vi "Set Package Info To VIs - NIPKG.vi"(0 "Project Path":path, 1 "Top Level/Always Included VIs":path[](array[path]), 5 "NIPKG Build Spec Name (NIPKG)":string="NIPKG", 7 "Target Name (My Computer)":string="My Computer", 9 "Destination Path":path, 11 "error in":errorcluster, 12 "Files Generated By Build":path[](array[path])) -> (15 "error out":errorcluster)   [LabVIEW 2017, in "CL_G3_VIComponentBuilder.lvlib"]
doc: "<B>Package details</B>\nVI Component Builder - NIPKG - v1.0.0-21\n\nPackage Filename - vicomponentbuilder-nipkg-1.0.0-21.nipkg"
uses:
  CL_G3_VIComponentBuilder.lvlib
  Exports/NIPKG_LV/NIPKG_LV.lvclass
  <vilib>/LVH/i3 JSON/JSON Parsing/Get Object Parameter Files/Get Object Parameter - Object.vi
  <vilib>/LVH/i3 JSON/JSON Parsing/Get Object Parameter Files/Get Object Parameter - Boolean.vi
  <vilib>/xml/Load XML File.vi
  <vilib>/xml/Close Reference(Node).vi
  <vilib>/xml/NI_XML.lvlib
  <vilib>/LVH/i3 JSON/i3-json.lvlib
panel:
  out "String":string
  out "Progress":i32(slide) scale=-1.0..109.0
  out "Total":i32
  # "Adding Package details to VI description"
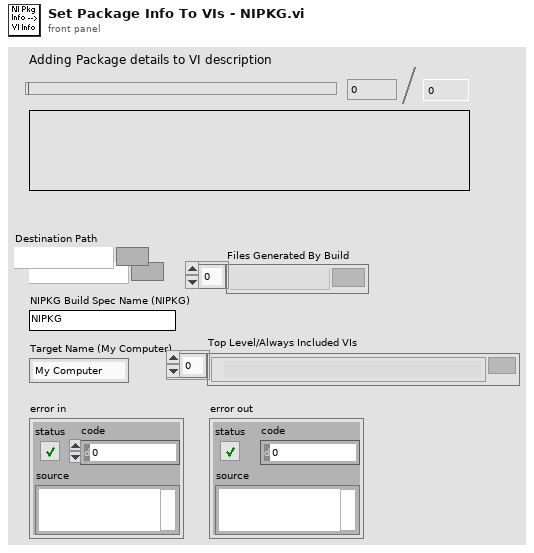
[diagram p1: front panel]
types:
  T1 = cluster{"Error State":errorcluster, "Processed Documentation":string, "Build Spec Path":path, "VIs In Package":path[], "Product Name":string, "Package Version":string, "Package Name":string, "Current File to process":path, "vi reference being processed":refnum<vi>, "Opened References":refnum<vi>[], "Build Options i3JSON Tree":variant}
  T2 = enum32{"Invalid", "Standard", "Closed", "Hidden", "Minimized", "Maximized"}
  T3 = cluster{"Beginning of Tag Position":i32, "End of Tag Position":i32}[]
  T4 = cluster{"Beginning of Tag Position":i32, "End of Tag Position":i32}
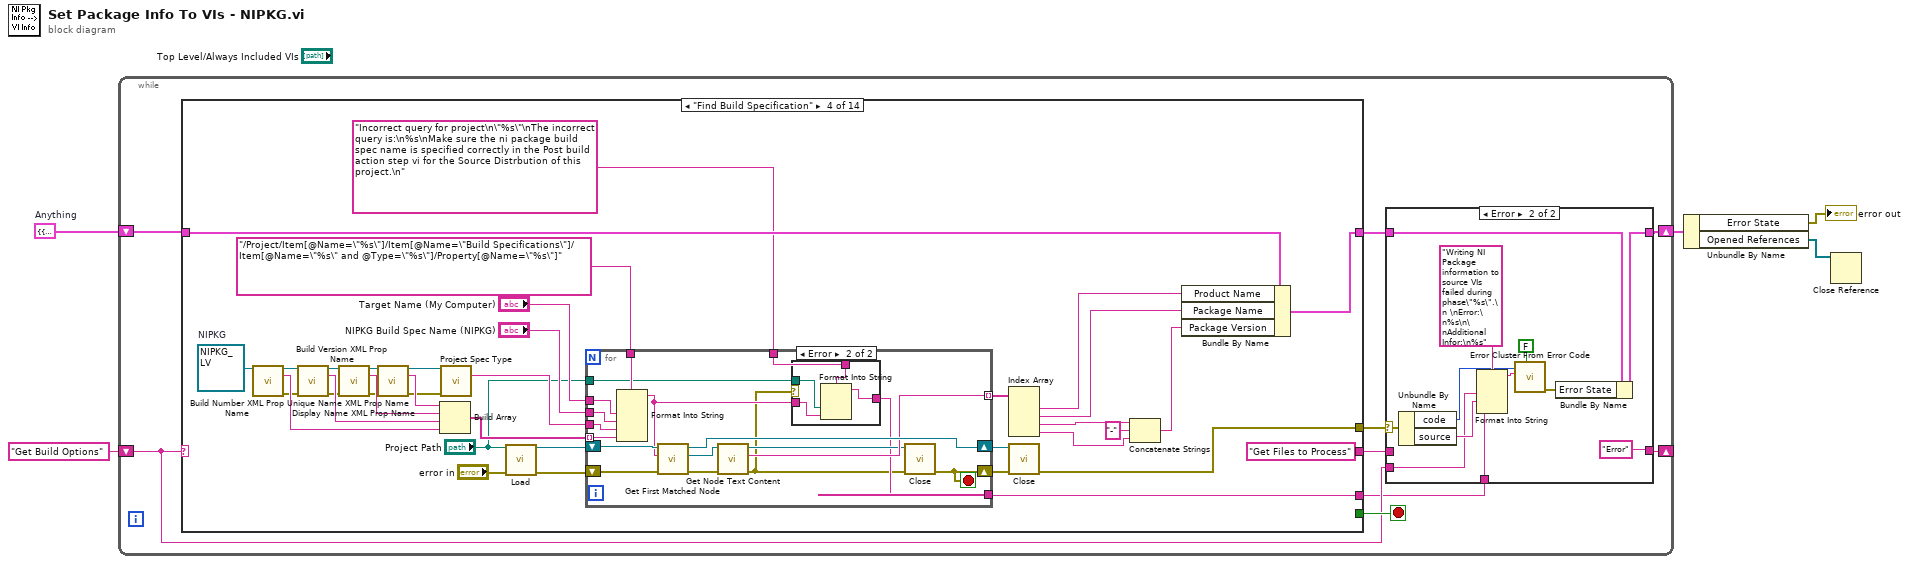
[diagram p0: block diagram]
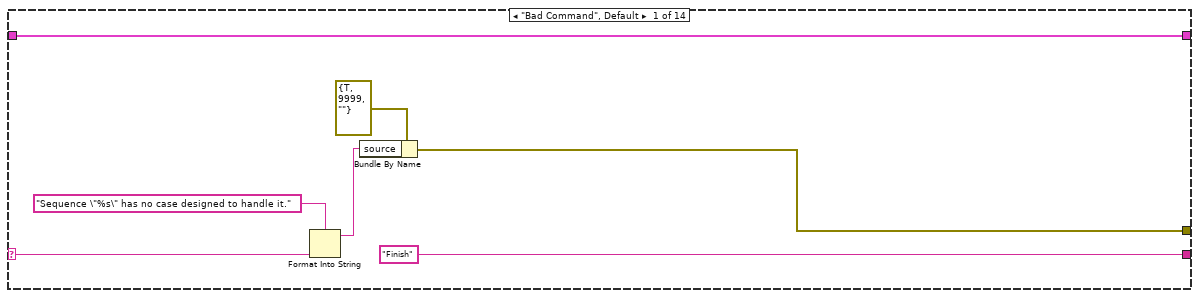
[diagram p3: hidden frame]
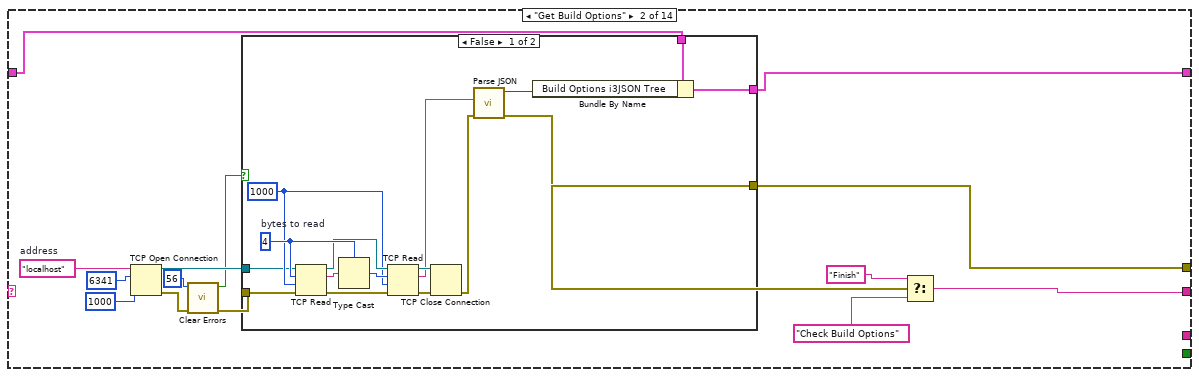
[diagram p4: hidden frame]
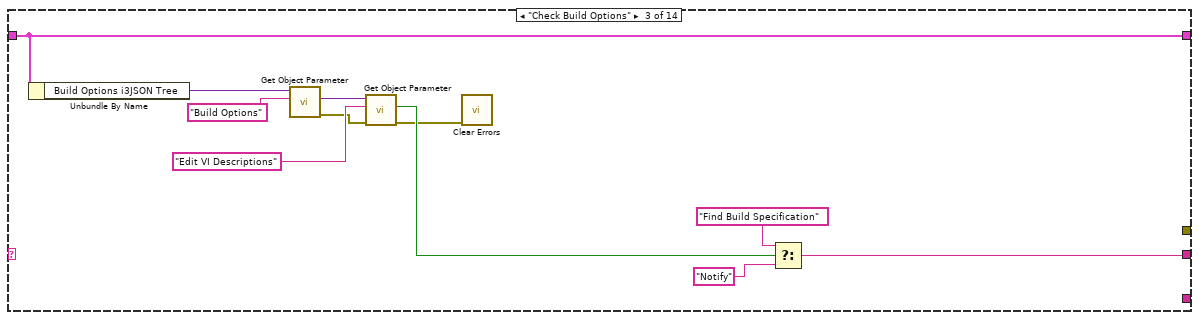
[diagram p6: hidden frame]
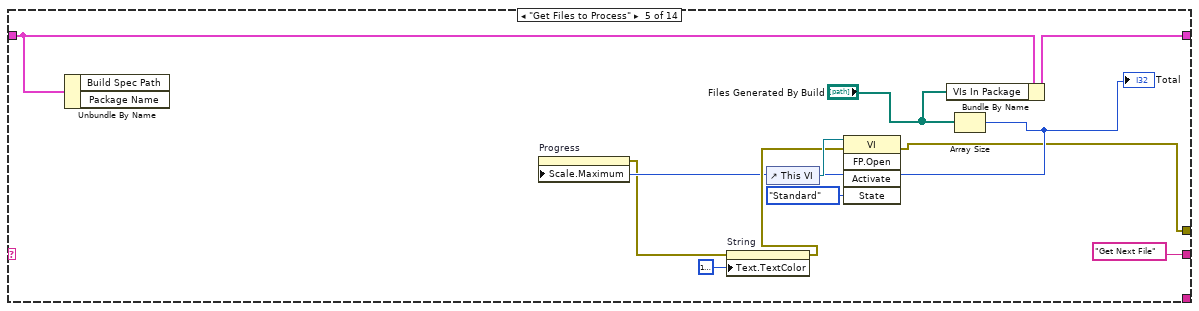
[diagram p8: hidden frame]
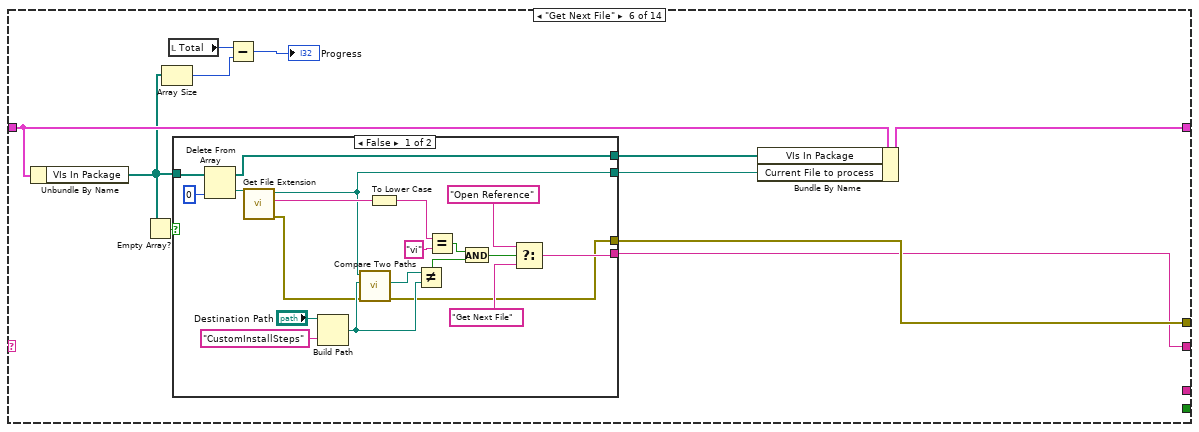
[diagram p9: hidden frame]
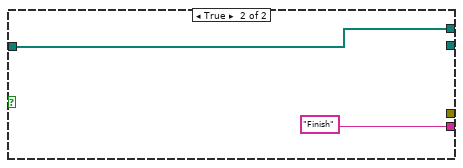
[diagram p10: hidden frame]
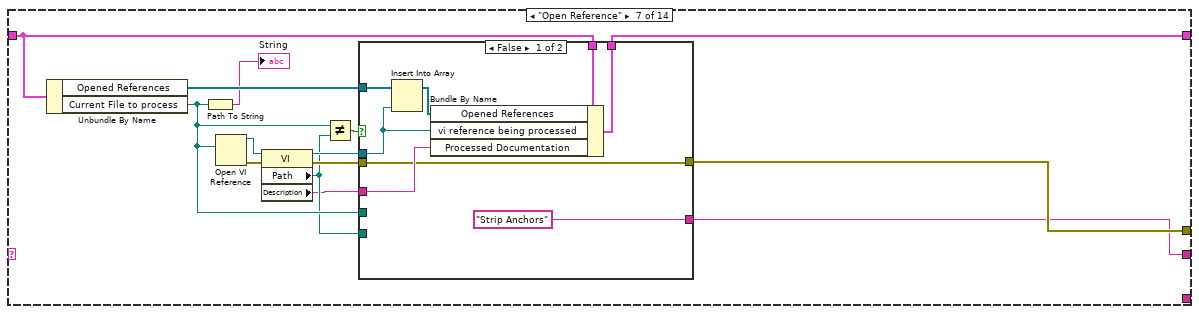
[diagram p11: hidden frame]
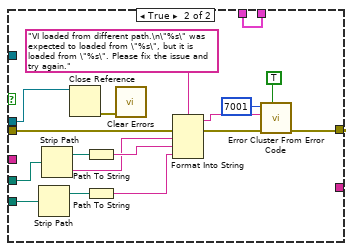
[diagram p12: hidden frame]
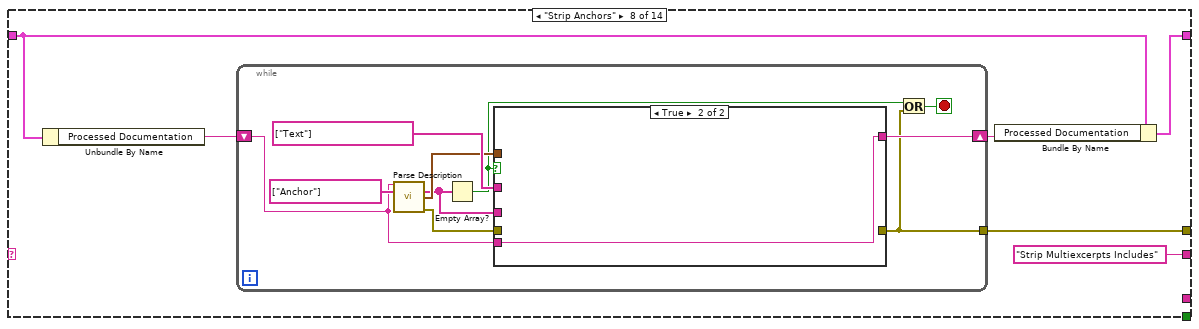
[diagram p13: hidden frame]
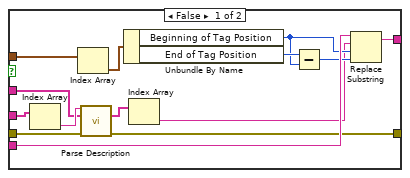
[diagram p14: hidden frame]
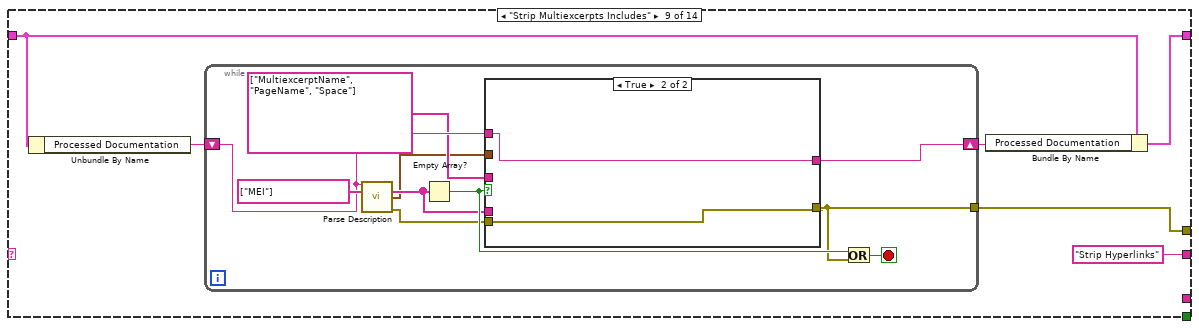
[diagram p15: hidden frame]
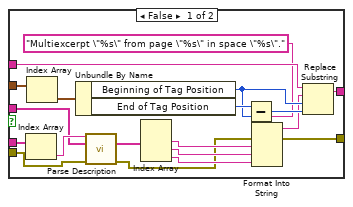
[diagram p16: hidden frame]
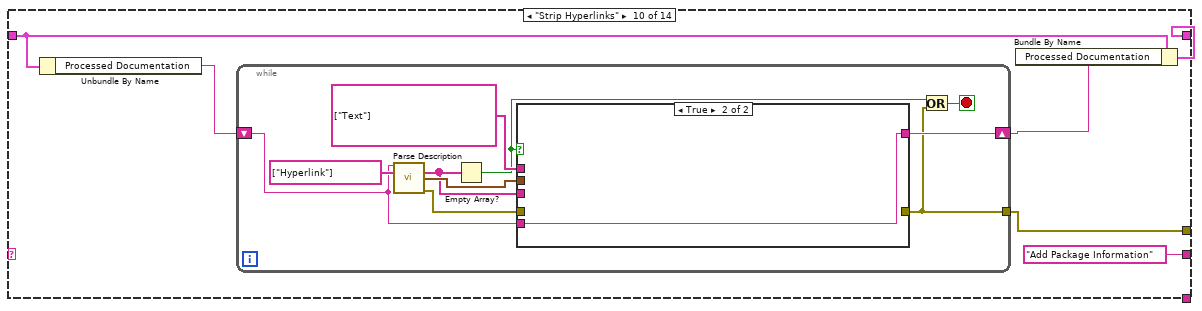
[diagram p17: hidden frame]
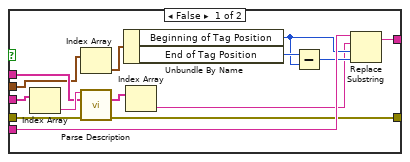
[diagram p18: hidden frame]
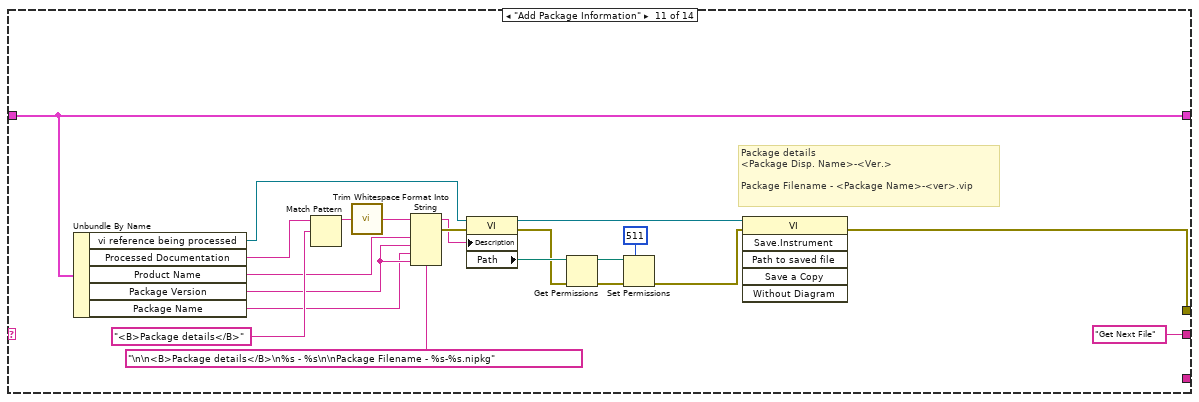
[diagram p19: hidden frame]
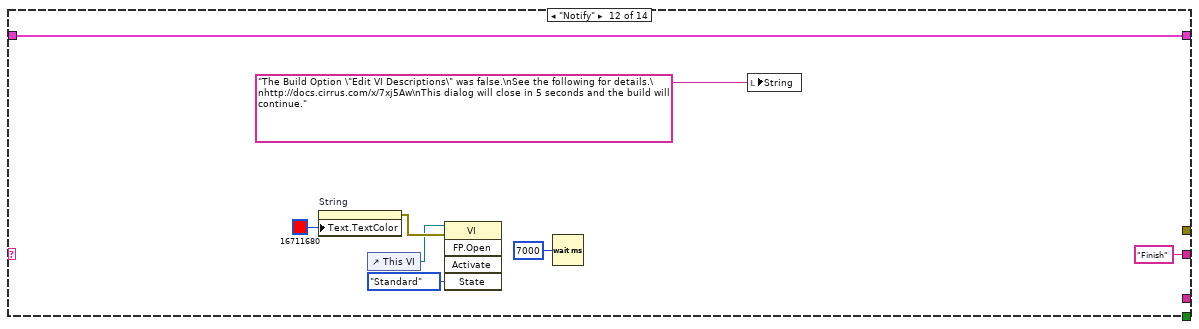
[diagram p20: hidden frame]
diagram:
  w3 = T1 {"Error State"={"status"=FALSE, "code"=0, "source"=""}, "Processed Documentation"="", "Build Spec Path"=path "", "VIs In Package"=[], "Product Name"="", "Package Version"="", "Package Name"="", "Current File to process"=path "", "vi reference being processed"=refnum, "Opened References"=[], "Build Options i3JSON Tree"=variant}  # Anything
  n1 = while {
    shift-right: [w8] -> w5
    shift-left: w3 -> [w14]
    shift-right: [w10] -> _
    shift-left: "Get Build Options" -> [w9]
    stop <- w13 stop-if-true
    n2 = case shown="\"Find Build Specification\"" w9 {
      selector: w9 -> [w32 _ _ _ _ _ _ _ _ _ _ _ _ _]
      tunnel: w14 -> [w35 w49 w75 w114 w145 w159 w187 w226 w257 w294 w332 w348 w350 w353]
      tunnel: [w35 w42 w75 w115 w146 w158 w186 w224 w255 w292 w332 w348 w350 w353] -> w12
      tunnel: ["Finish" ("Accessors:Name") w48 w76 "Get Files to Process" ("y") "Get Next File" w154 w185 "Strip Multiexcerpts Includes" ("y") "Strip Hyperlinks" ("y") "Add Package Information" ("y") "Get Next File" ("y") "Finish" ("y") "Finish" "Finish"] -> w11
      tunnel: [w30 w41 _ w98 w138 w156 w190 w222 w252 w289 w327 _ _ _] -> w7
      tunnel: [_ _ _ _ _ _ _ _ _ _ _ _ _ TRUE] -> w13
      tunnel: [_ _ _ w81 _ _ _ _ _ _ _ _ _ _] -> w6
      frame "Bad Command", Default {
        n3 = Format Into String(format string="Sequence \"%s\" has no case designed to handle it.", w32) -> (resulting string=w31:string)  [unwired: 2 in, 1 out]
        n4 = Bundle By Name(cluster=errorcluster {"status"=TRUE, "code"=9999, "source"=""} ("error out"), "source"=w31) -> (w30:errorcluster)
      }
      frame "Get Build Options" {
        w47 = "localhost"  # address
        n5 = TCP Open Connection(address=w47, remote port or service name=u16 6341, timeout ms (60000)=1000) -> (connection ID=w45:refnum<k5>, error out=w44:errorcluster)  [unwired: 2 in]
        n6 = call <vilib>:"Clear Errors.vi"("error in (no error)"=w44, "specific error code to clear (0: all)"=56) -> ("error out"=w38:errorcluster, "specific error cleared?"=w36:bool)  [unwired: 4 in]
        n7 = case shown="False" w36 {
          tunnel: w49 -> [w65 w66]
          tunnel: w45 -> [w58 _]
          tunnel: [w54 w66] -> w42
          tunnel: [w51 w67] -> w41
          tunnel: w38 -> [w50 w67]
          frame False {
            w59 = 1000 ("timeout ms (25000)")
            w63 = 4  # bytes to read
            n8 = TCP Read(connection ID=w58, bytes to read=w63, error in (no error)=w50, 9:w59) -> (connection ID out=w62:refnum<k5>, data out=w64:string, error out=w61:errorcluster)  [unwired: 1 in]
            n9 = Type Cast(type=w63, x=w64) -> (*(type *) &x=w60:i32)
            n10 = TCP Read(connection ID=w62, bytes to read=w60, error in (no error)=w61, 9:w59) -> (connection ID out=w57:refnum<k5>, data out=w55:string, error out=w56:errorcluster)  [unwired: 1 in]
            n11 = TCP Close Connection(connection ID=w57, error in (no error)=w56) -> (error out=w52:errorcluster)  [unwired: 1 in, 1 out]
            n12 = call <vilib>:"Parse JSON.vi"("error in (no error)"=w52, "JSON String"=w55) -> ("error out"=w51:errorcluster, "JSON Tree"=w53:variant)  [unwired: 6 in, 2 out]
            n13 = Bundle By Name(cluster=w65, "Build Options i3JSON Tree"=w53) -> (w54:T1)
          }
          frame True {
          }
        }
        n14 = Select(t="Finish", s=w41, f="Check Build Options") -> (s? t:f=w48:string)
      }
      frame "Check Build Options" {
        n15 = Unbundle By Name(w75) -> ("Build Options i3JSON Tree"=w74:variant)
        n16 = call-poly <vilib>:"Get Object Parameter.vi"("Parameter Name"="Build Options", "JSON Tree In (JSON Object)"=w74) -> ("error out"=w69:errorcluster, "JSON Object"=w73:variant)  [unwired: 6 in, 2 out]
        n17 = call-poly <vilib>:"Get Object Parameter.vi"("error in (no error)"=w69, "Parameter Name"="Edit VI Descriptions" ("Option Name"), "JSON Tree In (JSON Object)"=w73) -> ("error out"=w68:errorcluster, "Boolean Value"=w70:bool)  [unwired: 5 in, 2 out]
        n18 = call <vilib>:"Clear Errors.vi"("error in (no error)"=w68) -> ()  [unwired: 5 in, 2 out]
        n19 = Select(t="Find Build Specification", s=w70, f="Notify") -> (s? t:f=w76:string)
      }
      frame "Find Build Specification" {
        w84 = refnum<class "NIPKG_LV.lvclass"> refnum  # NIPKG
        n20 = call-dynamic "Build Number XML Prop Name.vi"("NI Build Specification in"=w84) -> ("NI Build Specification out"=w92:refnum<class "NIPKG_LV.lvclass">, "Build Number XML Property Name"=w93:string, "error out"=w91:errorcluster)  [unwired: 12 in]
        n21 = call-dynamic "Build Version XML Prop Name.vi"("NIPKG in"=w92, "error in (no error)"=w91) -> ("NIPKG out"=w90:refnum<class "NIPKG_LV.lvclass">, "Version Number XML Prop Name"=w94:string, "error out"=w89:errorcluster)  [unwired: 11 in]
        n22 = call-dynamic "Display Name XML Prop Name.vi"("NI Build Specification in"=w90, "error in (no error)"=w89) -> ("NI Build Specification out"=w88:refnum<class "NIPKG_LV.lvclass">, "Display Name XML Property Name"=w95:string, "error out"=w87:errorcluster)  [unwired: 11 in]
        n23 = call-dynamic "Unique Name XML Prop Name.vi"("NI Build Specification in"=w88, "error in (no error)"=w87) -> ("NI Build Specification out"=w86:refnum<class "NIPKG_LV.lvclass">, "Unique Name XML Property Name"=w96:string, "error out"=w85:errorcluster)  [unwired: 11 in]
        n24 = Build Array(w96, w95, w94, w93) -> (w83:string[])
        n25 = call-dynamic "Project Spec Type.vi"("NI Build Specification in"=w86, "error in (no error)"=w85) -> ("Project Specfication Type"=w82:string)  [unwired: 11 in, 2 out]
        n26 = call-poly <vilib>:"Load.vi"("path to XML document"="Project Path", "error in (no error)"="error in") -> ("DOM document out"=w111:refnum<k20>, "error out"=w106:errorcluster)  [unwired: 11 in, 1 out]
        n27 = for {
          tunnel: "/Project/Item[@Name=\"%s\"]/Item[@Name=\"Build Specifications\"]/Item[@Name=\"%s\" and @Type=\"%s\"]/Property[@Name=\"%s\"]" ("XPath expression") -> [w133]
          tunnel: w82 -> [w132]
          tunnel: "NIPKG Build Spec Name (NIPKG)" -> [w131]
          tunnel: w83 -> [w130] mode=indexing
          shift-right: [w128] -> w110
          shift-left: w111 -> [w129]
          tunnel: [w126] -> w105 mode=indexing
          shift-right: [w120] -> w109
          shift-left: w106 -> [w124]
          tunnel: "Target Name (My Computer)" -> [w123]
          tunnel: [w119] -> w81
          tunnel: "Incorrect query for project\n\"%s\"\nThe incorrect query is:\n%s\nMake sure the ni package build spec name is specified correctly in the Post build action step vi for the Source Distrbution of this project.\n" ("string") -> [w118]
          tunnel: "Project Path" -> [w117]
          stop <- w120 stop-if-true
          n28 = Format Into String(format string=w133, w123, w131, w132, w130) -> (resulting string=w121:string)  [unwired: 2 in, 1 out]
          n29 = call <vilib>:"Get First Matched Node.vi"("error in (no error)"=w124, "XPath expression"=w121, "node in"=w129) -> ("error out"=w122:errorcluster, "node result"=w127:refnum<k20>, "node out"=w128:refnum<k20>)  [unwired: 6 in]
          n30 = call <vilib>:"Get Node Text Content.vi"("error in (no error)"=w122, "node in"=w127) -> ("error out"=w116:errorcluster, "node text"=w126:string, "node out"=w125:refnum<k20>)  [unwired: 7 in]
          n31 = case shown="Error" w116 {
            tunnel: w121 -> [_ w136]
            tunnel: [_ w134] -> w119
            tunnel: w118 -> [_ w137]
            tunnel: w117 -> [_ w135]
            frame No Error {
            }
            frame Error {
              n32 = Format Into String(format string=w137, w135, w136) -> (resulting string=w134:string)  [unwired: 2 in, 1 out]
            }
          }
          n33 = call-poly <vilib>:"Close.vi"("error in (no error)"=w116, "node"=w125) -> ("error out"=w120:errorcluster)  [unwired: 7 in]
        }
        n34 = Index Array(array=w105) -> (element #1=w101:string, element #2=w100:string, element #3=w104:string, element #4=w103:string)  [unwired: 4 in]
        n35 = call-poly <vilib>:"Close.vi"("error in (no error)"=w109, "node"=w110) -> ("error out"=w98:errorcluster)  [unwired: 7 in]
        n36 = Concatenate Strings(w104, "-" ("string"), w103) -> (w99:string)
        n37 = Bundle By Name(cluster=w114, "Product Name"=w101, "Package Name"=w100, "Package Version"=w99) -> (w115:T1)
      }
      frame "Get Files to Process" {
        n38 = Unbundle By Name(w145) -> ()  [unwired: 2 out]
        n39 = control-ref of="This VI"() -> (w147:refnum<vi>)
        n40 = Bundle By Name(cluster=w145, "VIs In Package"="Files Generated By Build") -> (w146:T1)
        n41 = Array Size(array="Files Generated By Build") -> (size(s)=w140:i32)
        "Total" <- w140
        n42 = property on="Progress" class="Slide (strict)"("Scale.Maximum"=w140) -> (error out=w139:errorcluster)  [unwired: 2 in, 1 out]
        n43 = property on="String" class="Str"(error in=w139, "Text.TextColor"=u32 16777222) -> (error out=w141:errorcluster)  [unwired: 1 in, 1 out]
        n44 = invoke class="VI" method="FP.Open"(reference=w147, error in=w141, "State"=T2."Standard") -> (error out=w138:errorcluster)  [unwired: 2 in, 4 out]
      }
      frame "Get Next File" {
        n45 = Unbundle By Name(w159) -> ("VIs In Package"=w152:path[])
        n46 = Empty Array?(array=w152) -> (empty?=w155:bool)
        n47 = Array Size(array=w152) -> (size(s)=w151:i32)
        n48 = local read "Total"() -> (w150:i32)
        n49 = case shown="False" w155 {
          tunnel: [w165 _] -> w157
          tunnel: [w160 _] -> w156
          tunnel: w152 -> [w174 w180]
          tunnel: [w170 "Finish" ("y")] -> w154
          tunnel: [w169 w180] -> w153
          frame False {
            n50 = Delete From Array(array=w174, index=0) -> (deleted portion=w179:path, array with subset deleted=w169:path[])  [unwired: 1 in]
            n51 = call <vilib>:"Get File Extension.vi"("file"=w179) -> ("error out"=w161:errorcluster, "lowercase file extension"=w178:string, "dup file"=w165:path)  [unwired: 6 in, 2 out]
            n52 = Build Path(base path="Destination Path", name or relative path="CustomInstallSteps" ("regular expression")) -> (appended path=w163:path)
            n53 = call <vilib>:"Compare Two Paths.vi"("error in (no error)"=w161, "Path 2"=w163, "Path 1"=w165) -> ("error out"=w160:errorcluster, "Common Path"=w164:path)  [unwired: 5 in, 2 out]
            n54 = To Lower Case(string=w178) -> (all lower case string=w176:string)
            n55 = Not Equal?(x=w164, y=w163) -> (x != y?=w162:bool)
            n56 = Equal?(x=w176, y="vi") -> (x = y?=w175:bool)
            n57 = And(x=w175, y=w162) -> (x .and. y?=w173:bool)
            n58 = Select(t="Open Reference" ("y"), s=w173, f="Get Next File" ("y")) -> (s? t:f=w170:string)
          }
          frame True {
          }
        }
        n59 = Subtract(x=w150, y=w151) -> (x-y=→"Progress":i32)
        n60 = Bundle By Name(cluster=w159, "VIs In Package"=w153, "Current File to process"=w157) -> (w158:T1)
      }
      frame "Open Reference" {
        n61 = Unbundle By Name(w187) -> ("Opened References"=w183:refnum<vi>[], "Current File to process"=w189:path)
        n62 = Path To String(path=w189) -> (string=→"String":string)
        n63 = Open VI Reference(vi path=w189) -> (vi reference=w195:refnum<vi>, error out=w194:errorcluster)  [unwired: 5 in]
        n64 = property class="VI"(reference=w195, error in=w194) -> (reference out=w192:refnum<vi>, error out=w191:errorcluster, "Path"=w188:path, "Description"=w184:string)
        n65 = Not Equal?(x=w189, y=w188) -> (x != y?=w193:bool)
        n66 = case shown="False" w193 {
          tunnel: w192 -> [w198 w206]
          tunnel: w191 -> [w196 w210]
          tunnel: [w196 w209] -> w190
          tunnel: w189 -> [_ w208]
          tunnel: w188 -> [_ w207]
          tunnel: w187 -> [w203 w204]
          tunnel: [w202 w204] -> w186
          tunnel: ["Strip Anchors" _] -> w185
          tunnel: w184 -> [w200 _]
          tunnel: w183 -> [w199 _]
          frame False {
            n67 = Insert Into Array(array=w199, new element=w198) -> (w197:refnum<vi>[])  [unwired: 1 in]
            n68 = Bundle By Name(cluster=w203, "Opened References"=w197, "vi reference being processed"=w198, "Processed Documentation"=w200) -> (w202:T1)
          }
          frame True {
            n69 = Strip Path(path=w207) -> (stripped path=w216:path)  [unwired: 1 out]
            n70 = Strip Path(path=w208) -> (stripped path=w214:path, name=w213:string)
            n71 = Close Reference(reference=w206) -> (error out=w205:errorcluster)  [unwired: 1 in]
            n72 = Path To String(path=w214) -> (string=w215:string)
            n73 = Path To String(path=w216) -> (string=w217:string)
            n74 = call <vilib>:"Clear Errors.vi"("error in (no error)"=w205) -> ()  [unwired: 5 in, 2 out]
            n75 = Format Into String(format string="VI loaded from different path.\n\"%s\" was expected to loaded from \"%s\", but it is loaded from \"%s\". Please fix the issue and try again.", error in=w210, w213, w215, w217) -> (resulting string=w218:string, error out=w211:errorcluster)  [unwired: 1 in]
            n76 = call <vilib>:"Error Cluster From Error Code.vi"("show call chain? (False)"=TRUE, "error in (no error)"=w211, "error message (\"\")"=w218, "error code (0)"=7001) -> ("error out"=w209:errorcluster)  [unwired: 5 in]
          }
        }
      }
      frame "Strip Anchors" {
        n77 = Unbundle By Name(w226) -> ("Processed Documentation"=w225:string)
        n78 = while {
          shift-right: [w232] -> w223
          shift-left: w225 -> [w233]
          tunnel: [w229] -> w222
          stop <- w227 stop-if-true
          n79 = call "Parse Description.vi"("Description"=w233, "XML Values to Parse"=string[] ["Anchor"]) -> ("XML Values"=w230:string[], "String Bounds of Matches"=w234:T3, "error out"=w231:errorcluster)  [unwired: 10 in, 1 out]
          n80 = Empty Array?(array=w230) -> (empty?=w228:bool)
          n81 = case shown="True" w228 {
            tunnel: w230 -> [w250 _]
            tunnel: w231 -> [w247 _]
            tunnel: string[] ["Text"] ("XML Values to Parse") -> [w246 _]
            tunnel: w234 -> [w245 _]
            tunnel: w233 -> [w244 w251]
            tunnel: [w243 w251] -> w232
            tunnel: [w237 _] -> w229
            frame False {
              n82 = Index Array(array=w250) -> (element=w249:string)  [unwired: 1 in]
              n83 = Index Array(array=w245) -> (element=w242:T4)  [unwired: 1 in]
              n84 = call "Parse Description.vi"("Description"=w249, "XML Values to Parse"=w246, "error in (no error) 2"=w247) -> ("XML Values"=w248:string[], "error out"=w237:errorcluster)  [unwired: 9 in, 2 out]
              n85 = Unbundle By Name(w242) -> ("Beginning of Tag Position"=w240:i32, "End of Tag Position"=w241:i32)
              n86 = Index Array(array=w248) -> (element=w238:string)  [unwired: 1 in]
              n87 = Subtract(x=w241, y=w240) -> (x-y=w239:i32)
              n88 = Replace Substring(2:w239, 3:w240, 4:w238, 5:w244) -> (1:w243:string)  [unwired: 1 out]
            }
            frame True {
            }
          }
          n89 = Or(x=w228, y=w229) -> (x .or. y?=w227:bool)
        }
        n90 = Bundle By Name(cluster=w226, "Processed Documentation"=w223) -> (w224:T1)
      }
      frame "Strip Multiexcerpts Includes" {
        n91 = Unbundle By Name(w257) -> ("Processed Documentation"=w256:string)
        n92 = while {
          shift-right: [w265] -> w254
          shift-left: w256 -> [w266]
          tunnel: [w258] -> w252
          stop <- w263 stop-if-true
          n93 = call "Parse Description.vi"("Description"=w266, "XML Values to Parse"=string[] ["MEI"]) -> ("XML Values"=w262:string[], "String Bounds of Matches"=w260:T3, "error out"=w259:errorcluster)  [unwired: 10 in, 1 out]
          n94 = Empty Array?(array=w262) -> (empty?=w264:bool)
          n95 = case shown="True" w264 {
            tunnel: w260 -> [w286 _]
            tunnel: w266 -> [w285 w288]
            tunnel: [w284 w288] -> w265
            tunnel: w262 -> [w279 _]
            tunnel: string[] ["MultiexcerptName", "PageName", "Space"] ("XML Values to Parse") -> [w277 _]
            tunnel: [w269 w287] -> w258
            tunnel: w259 -> [w268 w287]
            frame False {
              n96 = Index Array(array=w279) -> (element=w278:string)  [unwired: 1 in]
              n97 = Index Array(array=w286) -> (element=w283:T4)  [unwired: 1 in]
              n98 = Unbundle By Name(w283) -> ("Beginning of Tag Position"=w281:i32, "End of Tag Position"=w282:i32)
              n99 = call "Parse Description.vi"("Description"=w278, "XML Values to Parse"=w277, "error in (no error) 2"=w268) -> ("XML Values"=w276:string[], "error out"=w270:errorcluster)  [unwired: 9 in, 2 out]
              n100 = Index Array(array=w276) -> (element #1=w275:string, element #2=w274:string, element #3=w273:string)  [unwired: 3 in]
              n101 = Subtract(x=w282, y=w281) -> (x-y=w280:i32)
              n102 = Format Into String(format string="Multiexcerpt \"%s\" from page \"%s\" in space \"%s\".", error in=w270, w275, w274, w273) -> (resulting string=w271:string, error out=w269:errorcluster)  [unwired: 1 in]
              n103 = Replace Substring(2:w280, 3:w281, 4:w271, 5:w285) -> (1:w284:string)  [unwired: 1 out]
            }
            frame True {
            }
          }
          n104 = Or(x=w264, y=w258) -> (x .or. y?=w263:bool)
        }
        n105 = Bundle By Name(cluster=w257, "Processed Documentation"=w254) -> (w255:T1)
      }
      frame "Strip Hyperlinks" {
        n106 = Unbundle By Name(w294) -> ("Processed Documentation"=w293:string)
        n107 = while {
          shift-right: [w300] -> w291
          shift-left: w293 -> [w301]
          tunnel: [w297] -> w289
          stop <- w296 stop-if-true
          n108 = call "Parse Description.vi"("Description"=w301, "XML Values to Parse"=string[] ["Hyperlink"]) -> ("XML Values"=w298:string[], "String Bounds of Matches"=w302:T3, "error out"=w299:errorcluster)  [unwired: 10 in, 1 out]
          n109 = Empty Array?(array=w298) -> (empty?=w295:bool)
          n110 = case shown="True" w295 {
            tunnel: w298 -> [w318 _]
            tunnel: w299 -> [w315 _]
            tunnel: string[] ["Text"] ("XML Values to Parse") -> [w314 _]
            tunnel: w302 -> [w313 _]
            tunnel: w301 -> [w312 w319]
            tunnel: [w311 w319] -> w300
            tunnel: [w305 _] -> w297
            frame False {
              n111 = Index Array(array=w318) -> (element=w317:string)  [unwired: 1 in]
              n112 = Index Array(array=w313) -> (element=w310:T4)  [unwired: 1 in]
              n113 = call "Parse Description.vi"("Description"=w317, "XML Values to Parse"=w314, "error in (no error) 2"=w315) -> ("XML Values"=w316:string[], "error out"=w305:errorcluster)  [unwired: 9 in, 2 out]
              n114 = Unbundle By Name(w310) -> ("Beginning of Tag Position"=w308:i32, "End of Tag Position"=w309:i32)
              n115 = Index Array(array=w316) -> (element=w306:string)  [unwired: 1 in]
              n116 = Subtract(x=w309, y=w308) -> (x-y=w307:i32)
              n117 = Replace Substring(2:w307, 3:w308, 4:w306, 5:w312) -> (1:w311:string)  [unwired: 1 out]
            }
            frame True {
            }
          }
          n118 = Or(x=w295, y=w297) -> (x .or. y?=w296:bool)
        }
        n119 = Bundle By Name(cluster=w294, "Processed Documentation"=w291) -> (w292:T1)
      }
      frame "Add Package Information" {
        # "Package details\n<Package Disp. Name>-<Ver.>\n\nPackage Filename - <Package Name>-<ver>.vip"
        n120 = Unbundle By Name(w332) -> ("vi reference being processed"=w326:refnum<vi>, "Processed Documentation"=w331:string, "Product Name"=w330:string, "Package Version"=w329:string, "Package Name"=w328:string)
        n121 = Match Pattern(string=w331, regular expression="<B>Package details</B>") -> (before substring=w335:string)  [unwired: 1 in, 3 out]
        n122 = call <vilib>:"Trim Whitespace.vi"("string"=w335) -> ("trimmed string"=w334:string)  [unwired: 1 in]
        n123 = Format Into String(format string="\n\n<B>Package details</B>\n%s - %s\n\nPackage Filename - %s-%s.nipkg", initial string=w334, w330, w329, w328, w329) -> (resulting string=w338:string, error out=w339:errorcluster)  [unwired: 1 in]
        n124 = property class="VI"(reference=w326, error in=w339, "Description"=w338) -> (reference out=w337:refnum<vi>, error out=w321:errorcluster, "Path"=w322:path)
        n125 = Get Permissions(8:w321, 11:w322) -> (0:w324:errorcluster, 3:w325:path)  [unwired: 3 out]
        n126 = Set Permissions(7:i16 511 ("permissions"), 8:w324, 11:w325) -> (0:w320:errorcluster)  [unwired: 2 in, 1 out]
        n127 = invoke class="VI" method="Save.Instrument"(reference=w337, error in=w320) -> (error out=w327:errorcluster)  [unwired: 4 in, 5 out]
      }
      frame "Notify" {
        n128 = property on="String" class="Str"("Text.TextColor"=u32 16711680) -> (error out=w347:errorcluster)  [unwired: 2 in, 1 out]
        n129 = control-ref of="This VI"() -> (w344:refnum<vi>)
        n130 = invoke class="VI" method="FP.Open"(reference=w344, error in=w347, "State"=T2."Standard") -> ()  [unwired: 2 in, 5 out]
        n131 = Wait (ms)(milliseconds to wait=u32 7000) -> ()  [unwired: 1 out]
        n132 = local write "String"("The Build Option \"Edit VI Descriptions\" was false.\nSee the following for details.\nhttp://docs.cirrus.com/x/7xj5Aw\nThis dialog will close in 5 seconds and the build will continue." ("String")) -> ()
      }
      frame "Error" {
      }
      frame "Finish" {
      }
    }
    n133 = case shown="Error" w7 {
      selector: w7 -> [_ w26]
      tunnel: [w16 w24] -> w8
      tunnel: w12 -> [w16 w25]
      tunnel: w9 -> [_ w21]
      tunnel: [w15 "Error"] -> w10
      tunnel: w11 -> [w15 _]
      tunnel: w6 -> [_ w17]
      frame No Error {
      }
      frame Error {
        n134 = Unbundle By Name(w26) -> ("code"=w20:i32, "source"=w22:string)
        n135 = Format Into String(format string="Writing NI Package information to source VIs failed during phase\"%s\".\n \nError:\n%s\n\nAdditional Infor:\n%s" ("error message (\"\")"), w21, w22, w17) -> (resulting string=w27:string)  [unwired: 2 in, 1 out]
        n136 = call <vilib>:"Error Cluster From Error Code.vi"("show call chain? (False)"=FALSE, "error message (\"\")"=w27, "error code (0)"=w20) -> ("error out"=w18:errorcluster)  [unwired: 6 in]
        n137 = Bundle By Name(cluster=w25, "Error State"=w18) -> (w24:T1)
      }
    }
  }
  n138 = Unbundle By Name(w5) -> ("Error State"=→"error out":errorcluster, "Opened References"=w2:refnum<vi>[])
  n139 = Close Reference(reference=w2) -> ()  [unwired: 1 in, 1 out]
